vi "Write Value.vi"(8 "error in (no error)":errorcluster, 10 "Value":string, 11 "String D Element in":refnum<class "String D Element.lvclass">) -> (0 "error out":errorcluster, 3 "String D Element out":refnum<class "String D Element.lvclass">)   [LabVIEW 2018, in "D Datagrid Library.lvlib" / "String D Element.lvclass"]
uses:
  String D Element.lvclass
  String D Element.lvclass/String D Element.ctl
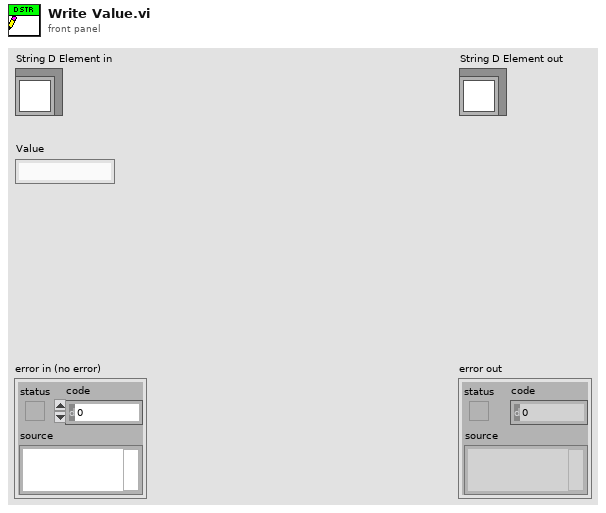
[diagram p1: front panel]
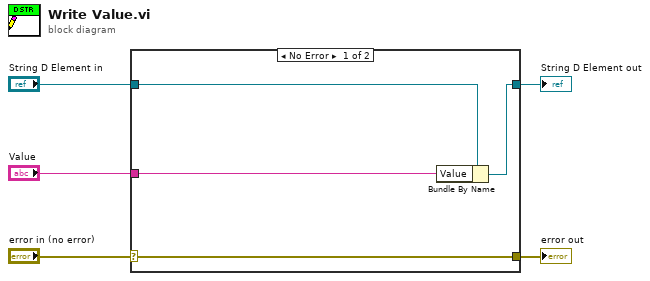
[diagram p0: block diagram]
diagram:
  n1 = case shown="No Error" "error in (no error)" {
    selector: "error in (no error)" -> [w9 w10]
    tunnel: [w9 w10] -> w4
    tunnel: [w7 w11] -> w2
    tunnel: "String D Element in" -> [w8 w11]
    tunnel: "Value" -> [w6 _]
    frame No Error {
      n2 = Bundle By Name(cluster=w8, "Value"=w6) -> (w7:refnum<class "String D Element.lvclass">)
    }
    frame Error {
    }
  }
  "error out" <- w4
  "String D Element out" <- w2
